vi "Fibonacci.vi"() -> ()   [LabVIEW 2016]
panel:
  out "Output":i32
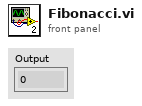
[diagram p1: front panel]
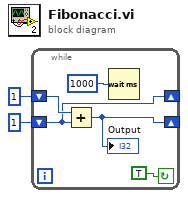
[diagram p0: block diagram]
diagram:
  n1 = while {
    shift-right: [w4] -> _
    shift-left: 1 -> [w6]
    shift-right: [w5] -> _
    shift-left: 1 -> [w4]
    stop <- TRUE continue-if-true
    n2 = Add(x=w6, y=w4) -> (x+y=w5:i32)
    "Output" <- w5
    n3 = Wait (ms)(milliseconds to wait=1000) -> ()  [unwired: 1 out]
  }
